vi "Read Waveform.vi"(8 "error in (no error)":errorcluster, 10 "# samples":i32, 11 "device handle in":T1) -> (0 "error out":errorcluster, 2 "Waveform":waveform(cdb), 3 "device handle out":T1)   [LabVIEW 2021, in "RTL-SDR.lvlib"]
uses:
  RTL-SDR.lvlib
  Controls/Device Handle.ctl
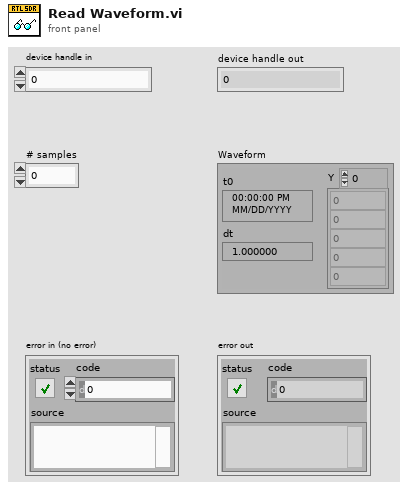
[diagram p1: front panel]
types:
  T1 = typedef "RTL-SDR.lvlib/Device Handle.ctl" = u64
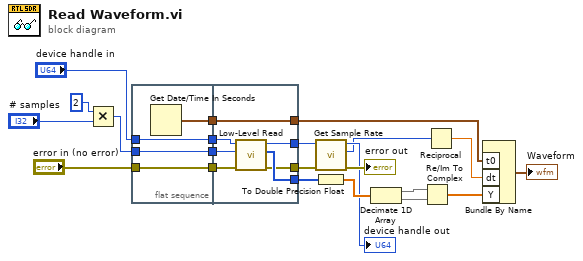
[diagram p0: block diagram]
diagram:
  n1 = Multiply(x=2, y="# samples") -> (x*y=w16:i32)
  n2 = flat-sequence {
    tunnel: "device handle in" -> [w24]
    tunnel: "error in (no error)" -> [w25]
    tunnel: w16 -> [w26]
    tunnel: [w26] -> w5
    tunnel: [w25] -> w4
    tunnel: [w24] -> w3
    tunnel: [w23] -> w1
    tunnel: [w33] -> w22
    tunnel: [w29] -> w13
    tunnel: [w28] -> w12
    tunnel: w5 -> [w32]
    tunnel: w4 -> [w31]
    tunnel: w3 -> [w30]
    tunnel: [w27] -> w2
    tunnel: w1 -> [w27]
    frame #0 {
      n3 = Get Date/Time In Seconds() -> (seconds since 1Jan1904=w23:timestamp)
    }
    frame #1 {
      n4 = call "Low-Level Read.vi"("error in (no error)"=w31, "# Samples to read"=w32, "device handle in"=w30) -> ("error out"=w28:errorcluster, "Samples"=w33:u8[], "device handle out"=w29:T1)  [unwired: 5 in, 1 out]
    }
  }
  n5 = call "Get Sample Rate.vi"("error in (no error)"=w12, "device handle in"=w13) -> ("error out"=→"error out":errorcluster, "Sample Rate (Hz)"=w9:u32, "device handle out"=→"device handle out":T1)  [unwired: 7 in]
  n6 = To Double Precision Float(number=w22) -> (double precision float=w19:dbl[])
  n7 = Decimate 1D Array(w19) -> (w20:dbl[], w21:dbl[])
  n8 = Re/Im To Complex(1:w21, 2:w20) -> (0:w7:cdb[])
  n9 = Reciprocal(x=w9) -> (1/x=w8:dbl)
  n10 = Bundle By Name("t0"=w2, "dt"=w8, "Y"=w7) -> (→"Waveform":waveform(cdb))  [unwired: 1 in]
